vi "Generate Waveform.vi"(1 "Index":i32) -> (0 "Waveform Point":dbl format="%.2f")   [LabVIEW 2012]
doc: "Generate Waveform.vi creates a point on a wave similar to a sinc function. The input is designed to be an index and the output is the sinc-like waves value at that point."
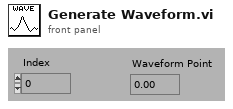
[diagram p1: front panel]
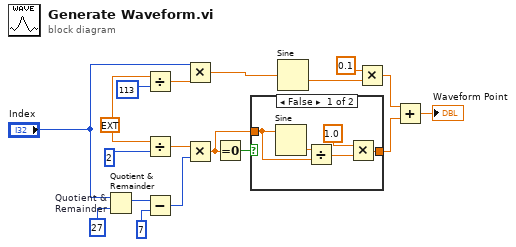
[diagram p0: block diagram]
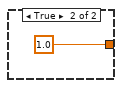
[diagram p2: hidden frame]
diagram:
  w18 = ext 3.1415926535897932385
  n1 = Quotient & Remainder "Quotient &\nRemainder"(x="Index", y=27) -> (x-y*floor(x/y)=w15:i32)  [unwired: 1 out]
  n2 = Divide(x=w18, y=113) -> (x/y=w9:ext)
  n3 = Divide(x=w18, y=2) -> (x/y=w13:ext)
  n4 = Subtract(x=w15, y=7) -> (x-y=w12:i32)
  n5 = Multiply(x="Index", y=w9) -> (x*y=w8:ext)
  n6 = Multiply(x=w13, y=w12) -> (x*y=w10:ext)
  n7 = Equal To 0?(x=w10) -> (x = 0?=w11:bool)
  n8 = case shown="False" w11 {
    tunnel: [w21 1.0] -> w4
    tunnel: w10 -> [w22 _]
    frame False {
      n9 = Sine(x=w22) -> (sin(x)=w23:ext)
      n10 = Divide(x=w23, y=w22) -> (x/y=w19:ext)
      n11 = Multiply(x=1.0, y=w19) -> (x*y=w21:ext)
    }
    frame True {
    }
  }
  n12 = Sine(x=w8) -> (sin(x)=w7:ext)
  n13 = Multiply(x=0.1, y=w7) -> (x*y=w5:ext)
  n14 = Add(x=w5, y=w4) -> (x+y=→"Waveform Point":ext)
